vi "VHM-sendConnectionStatus.vi"(8 "error in (no error)":errorcluster, 11 "VHM-VNA_Hardware_Manager in":refnum<class "VHM-VNA_Hardware_Manager.lvclass">) -> (0 "error out":errorcluster, 3 "VHM-VNA_Hardware_Manager out":refnum<class "VHM-VNA_Hardware_Manager.lvclass">)   [LabVIEW 2020, in "VHM-VNA_Hardware_Manager.lvlib" / "VHM-VNA_Hardware_Manager.lvclass"]
uses:
  VHM-VNA_Hardware_Manager.lvclass
  VHM-connection_status.ctl
  VHM-VNA_Hardware_Manager.lvclass/VHM-VNA_Hardware_Manager.ctl
  VHMI-VNA_Hardware_manager_Interface Messages/VHMI-recieveConnectionInfo Msg/VHMI-recieveConnectionInfo Msg.lvclass/VHMI-recieveConnectionInfo Msg.ctl
  <vilib>/ActorFramework/Message Enqueuer/Message Enqueuer.lvclass/Message Enqueuer.ctl
  <vilib>/ActorFramework/Message Enqueuer/Enqueue.vi
  VHMI-VNA_Hardware_manager_Interface Messages/VHMI-recieveConnectionInfo Msg/VHMI-recieveConnectionInfo Msg.lvclass
  C:/Program Files (x86)/National Instruments/LabVIEW 2020/vi.lib/ActorFramework/Message/Message.lvclass
  <vilib>/ActorFramework/Message Priority Queue/Priority Enqueue.vi
  classes/vna-drivers/liteVNA/VD-LV-LiteVNA.lvclass
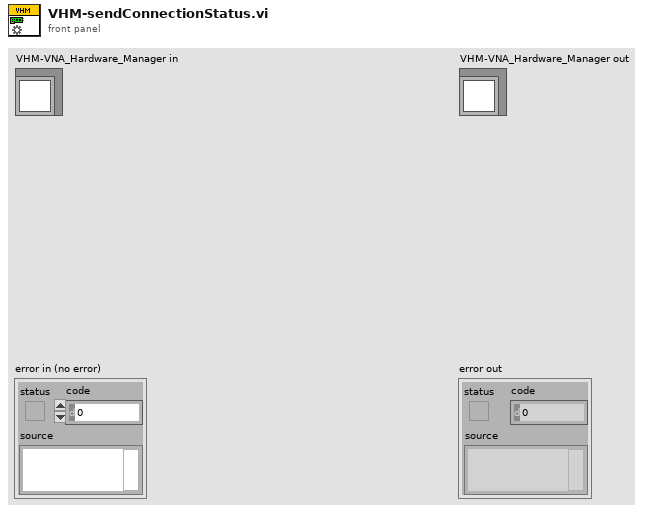
[diagram p1: front panel]
types:
  T1 = typedef "VHM-VNA_Hardware_Manager.lvlib/VHM-VNA_Hardware_Manager.lvclass/VHM-connection_status.ctl" = cluster{"Connected?":bool, "Status":string}
  T2 = typedef "VD-LV-LiteVNA.lvclass/VD-session_info.ctl" = cluster{"last set TS":timestamp, "last get TS":timestamp, "last set":T3, "last get":T3, "Connected?":bool}
  T3 = typedef "HP-S-Serial.lvclass/HP-S-data.ctl" = u8[]
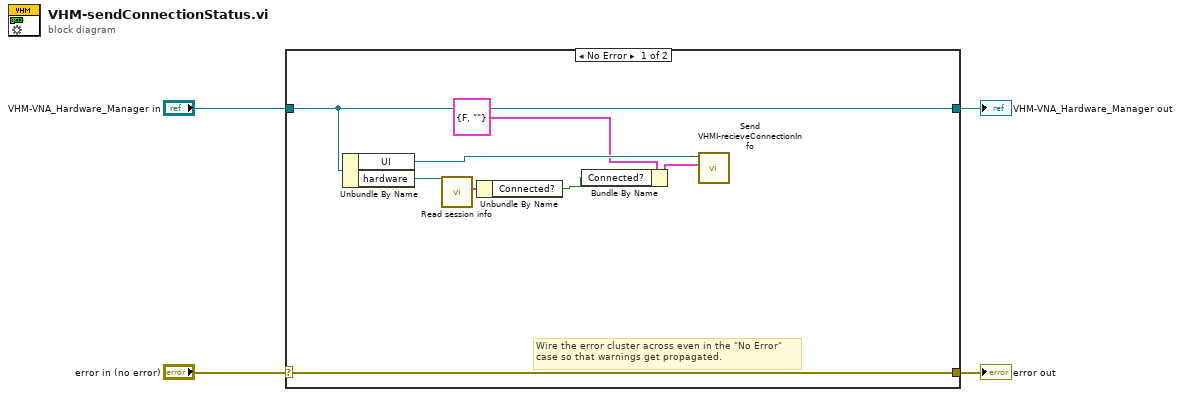
[diagram p0: block diagram]
diagram:
  n1 = case shown="No Error" "error in (no error)" {
    selector: "error in (no error)" -> [w11 w14]
    tunnel: [w11 w14] -> w3
    tunnel: [w12 w13] -> w1
    tunnel: "VHM-VNA_Hardware_Manager in" -> [w12 w13]
    frame No Error {
      # "Wire the error cluster across even in the \"No Error\"\ncase so that warnings get propagated."
      n2 = Unbundle By Name(w12) -> ("UI"=w10:refnum<class "Message Enqueuer.lvclass">, "hardware"=w9:refnum<class "VD-LV-LiteVNA.lvclass">)
      n3 = call-dynamic "Read session info.vi"("VD-LV-LiteVNA in"=w9) -> ("session info"=w6:T2)  [unwired: 8 in, 2 out]
      n4 = Unbundle By Name(w6) -> ("Connected?"=w5:bool)
      n5 = Bundle By Name(cluster=T1 {"Connected?"=FALSE, "Status"=""} ("connection status"), "Connected?"=w5) -> (w7:T1)
      n6 = call "Send VHMI-recieveConnectionInfo.vi"("connection status"=w7, "Message Enqueuer"=w10) -> ()  [unwired: 8 in, 2 out]
    }
    frame Error {
    }
  }
  "error out" <- w3
  "VHM-VNA_Hardware_Manager out" <- w1
